vi "EventClient_SubscribeEvents.vi"(8 "error in (no error)":errorcluster, 10 "Events":string[](array[string]), 11 "reference":T1) -> (0 "error out":errorcluster, 3 "reference out":T1)   [LabVIEW 2018]
uses:
  EventClient_ObjectReference.ctl
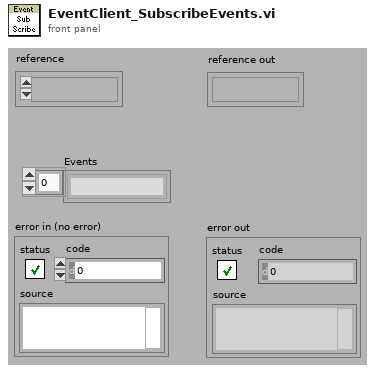
[diagram p1: front panel]
types:
  T1 = typedef "EventClient_ObjectReference.ctl" = refnum<k1>
  T2 = cluster{"Client":refnum<queue>, "Sub Events":string[], "PrvData":variant, "MyName":string}
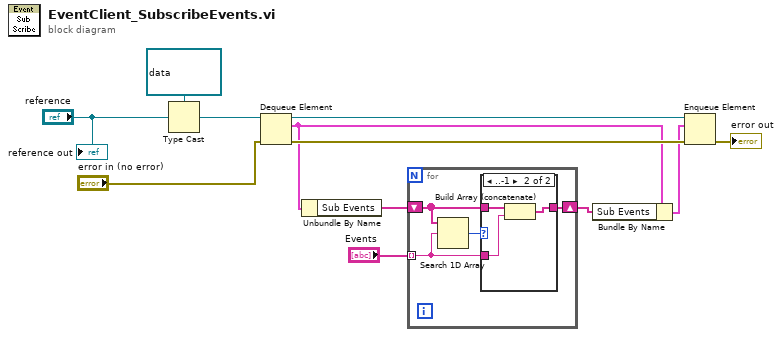
[diagram p0: block diagram]
diagram:
  n1 = Type Cast(type=refnum<queue> refnum ("queue out"), x="reference") -> (*(type *) &x=w11:refnum<queue>)
  n2 = Dequeue Element(queue=w11, error in (no error)="error in (no error)") -> (queue out=w8:refnum<queue>, element=w6:T2, error out=w7:errorcluster)  [unwired: 2 out]
  n3 = Unbundle By Name(w6) -> ("Sub Events"=w10:string[])
  n4 = for {
    tunnel: "Events" -> [w14] mode=indexing
    shift-right: [w16] -> w5
    shift-left: w10 -> [w15]
    n5 = Search 1D Array(1D array=w15, element=w14) -> (index of element=w13:i32)  [unwired: 1 out]
    n6 = case shown="..-1" w13 {
      tunnel: w15 -> [w17 w20]
      tunnel: w14 -> [_ w19]
      tunnel: [w17 w18] -> w16
      frame 0, Default {
      }
      frame ..-1 {
        n7 = Build Array (concatenate)(w20, w19) -> (w18:string[])
      }
    }
  }
  n8 = Bundle By Name(cluster=w6, "Sub Events"=w5) -> (w4:T2)
  n9 = Enqueue Element(queue=w8, element=w4, error in (no error)=w7) -> (error out=→"error out":errorcluster)  [unwired: 3 out]
  "reference out" <- "reference"
